vi "KalmanFilter_SetXHat.vi"(9 "xHat":T1, 11 "in KalmanFilter":T2) -> (3 "out KalmanFilter":T2)   [LabVIEW 2019, in "Trajectory_Library.lvlib"]
doc: "Creates a new LINEAR SYSTEM data cluster with the specified values. \n\n\nInputs: \n - XXX -- XXX.\n\nOutputs:\n - XXX -- XXX."
uses:
  KALMAN_FILTER.ctl
  <vilib>/Analysis/Matrix/Datatypes/RealMatrix.ctl
  LINEAR_SYSTEM.ctl
  Trajectory_Library.lvlib
  <vilib>/Analysis/Matrix/NI_Matrix.lvlib
panel:
  # "Steady State Gain  \n<States,Outputs>"
  # "State Estimate <Statess,1>"
  # "<States,States>"
  # "<States,Inputs>"
  # "<Outputs,States>"
  # "<Outputs,Inputs>"
  # "Steady State Gain  \n<States,Outputs>"
  # "State Estimate <Statess,1>"
  # "<States,States>"
  # "<States,Inputs>"
  # "<Outputs,States>"
  # "<Outputs,Inputs>"
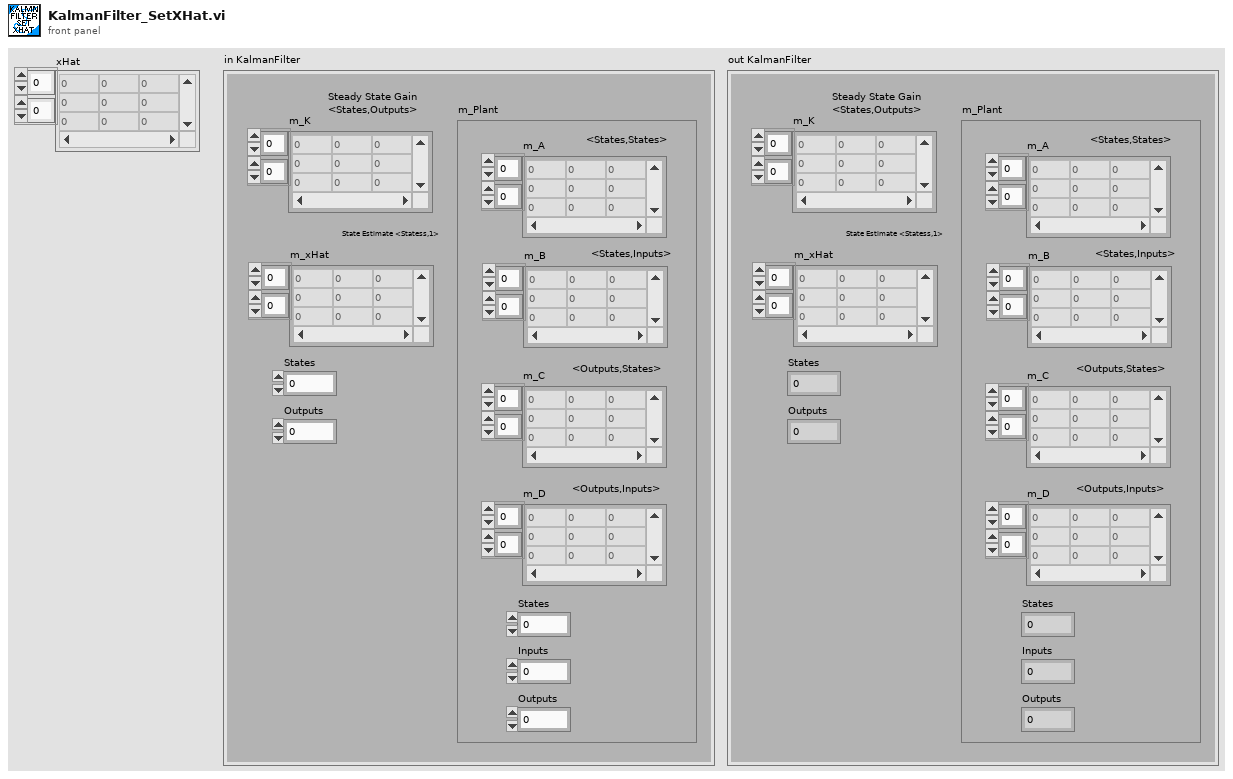
[diagram p1: front panel]
types:
  T1 = typedef "NI_Matrix.lvlib/RealMatrix.ctl" = dbl[][]
  T2 = typedef "Trajectory_Library.lvlib/KALMAN_FILTER.ctl" = cluster{"m_K":T1, "m_xHat":T1, "States":i32, "Outputs":i32, "m_Plant":T3}
  T3 = typedef "Trajectory_Library.lvlib/LINEAR_SYSTEM.ctl" = cluster{"m_A":T1, "m_B":T1, "m_C":T1, "m_D":T1, "States":i32, "Inputs":i32, "Outputs":i32}
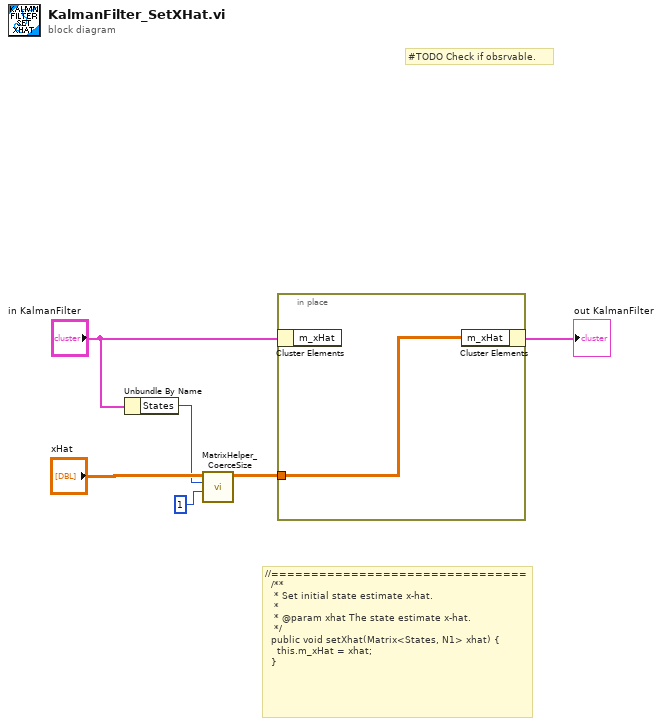
[diagram p0: block diagram]
diagram:
  # "//================================\n  /**\n   * Set initial state estimate x-hat.\n   *\n   * @param xhat The state estimate x-hat.\n   */\n  public void setXhat(Matrix<States, N1> xhat) {\n    this.m_xHat = xhat;\n  }"
  # "#TODO Check if obsrvable."
  n1 = Unbundle By Name("in KalmanFilter") -> ("States"=w2:i32)
  n2 = call "MatrixHelper_CoerceSize.vi"("Columns"=1, "Rows"=w2, "input matrix"="xHat") -> ("output matrix"=w3:T1)  [unwired: 8 in]
  n3 = in-place {
    in-place-border: w3 -> [w7]
    n4 = in-place-cluster #1("in KalmanFilter") -> ()  [unwired: 1 out]
    n5 = in-place-cluster #1("m_xHat"=w7) -> (→"out KalmanFilter":T2)
  }
